vi "GEA2 Script_Queue Info.vi"(0 "Script Info":T1={"Overall Script File Progress"=1.0, "Current Script Progress"=0.0, "Script"="", "Test"="", "Elapsed time (s)"=0.0, "Done?"=FALSE} {"Overall Script File Progress" scale=0.0..1.0; "Elapsed time (s)" format="%#.1f"; "Current Script Progress" scale=0.0..1.0}, 11 "error in (no error)":errorcluster) -> (15 "error out":errorcluster)   [LabVIEW 2023]
uses:
  typedefs/Script Info.ctl
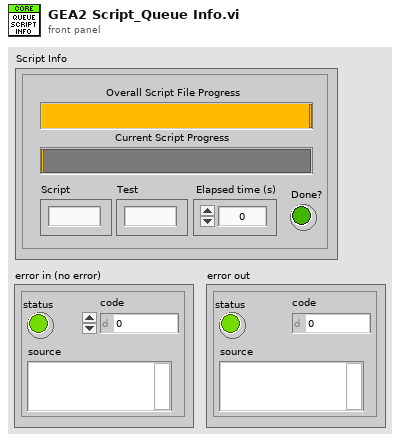
[diagram p1: front panel]
types:
  T1 = typedef "Script Info.ctl" = cluster{"Overall Script File Progress":dbl, "Current Script Progress":dbl, "Script":string, "Test":string, "Elapsed time (s)":dbl, "Done?":bool}
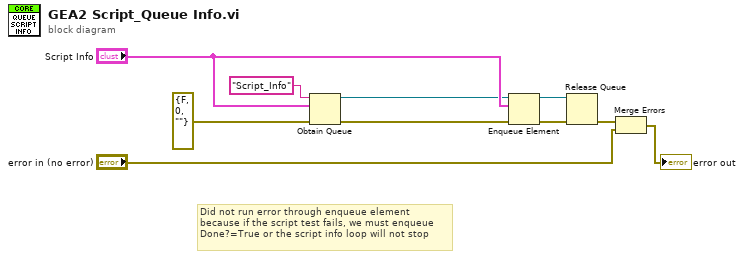
[diagram p0: block diagram]
diagram:
  # "Did not run error through enqueue element\nbecause if the script test fails, we must enqueue\nDone?=True or the script info loop will not stop"
  n1 = Obtain Queue(name (unnamed)="Script_Info", element data type="Script Info", error in (no error)=errorcluster {"status"=FALSE, "code"=0, "source"=""}) -> (queue out=w8:refnum<queue>, error out=w9:errorcluster)  [unwired: 2 in, 1 out]
  n2 = Enqueue Element(queue=w8, element="Script Info", error in (no error)=w9) -> (queue out=w5:refnum<queue>, error out=w6:errorcluster)  [unwired: 1 in, 1 out]
  n3 = Release Queue(queue=w5, error in (no error)=w6) -> (error out=w3:errorcluster)  [unwired: 1 in, 2 out]
  n4 = Merge Errors(w3, "error in (no error)") -> (→"error out":errorcluster)
